vi "Write Selection.vi"(8 "error in (no error)":errorcluster, 10 "Select Tags[]":string[](array[string]), 11 "TreeSelectionHierarchal in":refnum<class "TreeSelectionHierarchal.lvclass">) -> (0 "error out":errorcluster, 3 "TreeSelectionHierarchal out":refnum<class "TreeSelectionHierarchal.lvclass">)   [LabVIEW 2015, in "TreeSelectionHierarchal.lvclass"]
doc: "This property gets or sets the items which are selected (have the TRUE checkbox).\n<b> </b> <b> </b>\n©2016 Q Software Innovations, LLC (QSI)\nwritten by Quentin Alldredge\nproduced in LabVIEW 2015\n\nsupport@qsoftwareinnovations.com\nwww.qsoftwareinnovations.com\n\nAll rights reserved.\n\nRedistribution and use in source and binary forms, with or without modification, are permitted provided that the following conditions are met:\n\n * Redistributions of source code must retain the above copyright notice, this list of conditions and the following disclaimer.\n * Redistributions in binary form must reproduce the above copyright notice, this list of conditions and the following disclaimer in the documentation and/or other materials provided with the distribution.\n * Neither the name of Q Software Innovations, LLC. nor the names of its contributors may be used to endorse or promote products derived from this software without specific prior written permission.\n\nTHIS SOFTWARE IS PROVIDED BY THE COPYRIGHT HOLDERS AND CONTRIBUTORS \"AS IS\" AND ANY EXPRESS OR IMPLIED WARRANTIES, INCLUDING, BUT NOT LIMITED TO, THE IMPLIED WARRANTIES OF MERCHANTABILITY AND FITNESS FOR A PARTICULAR PURPOSE ARE DISCLAIMED. IN NO EVENT SHALL THE COPYRIGHT OWNER OR CONTRIBUTORS BE LIABLE FOR ANY DIRECT, INDIRECT, INCIDENTAL, SPECIAL, EXEMPLARY, OR CONSEQUENTIAL DAMAGES (INCLUDING, BUT NOT LIMITED TO, PROCUREMENT OF SUBSTITUTE GOODS OR SERVICES; LOSS OF USE, DATA, OR PROFITS; OR BUSINESS INTERRUPTION) HOWEVER CAUSED AND ON ANY THEORY OF LIABILITY, WHETHER IN CONTRACT, STRICT LIABILITY, OR TORT (INCLUDING NEGLIGENCE OR OTHERWISE) ARISING IN ANY WAY OUT OF THE USE OF THIS SOFTWARE, EVEN IF ADVISED OF THE POSSIBILITY OF SUCH DAMAGE."
uses:
  TreeSelectionHierarchal.lvclass
  TreeSelection/TreeSelection.lvclass
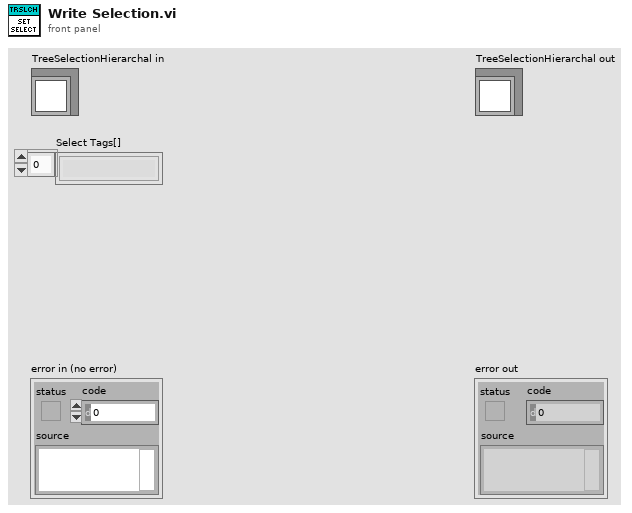
[diagram p1: front panel]
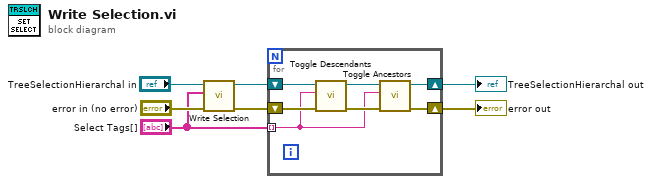
[diagram p0: block diagram]
diagram:
  n1 = call-parent "Write Selection.vi"("error in (no error)"="error in (no error)", "Selection[]"="Select Tags[]", "TreeSelection in"="TreeSelectionHierarchal in") -> ("error out"=w3:errorcluster, "TreeSelection out"=w5:refnum<class "TreeSelectionHierarchal.lvclass">)  [unwired: 7 in]
  n2 = for {
    shift-right: [w9] -> w4
    shift-left: w5 -> [w14]
    shift-right: [w11] -> w2
    shift-left: w3 -> [w13]
    tunnel: "Select Tags[]" -> [w8] mode=indexing
    n3 = call "Toggle Descendants.vi"("error in (no error)"=w13, "Tag"=w8, "TreeHier in"=w14) -> ("error out"=w12:errorcluster, "TreeHier out"=w10:refnum<class "TreeSelectionHierarchal.lvclass">)  [unwired: 7 in]
    n4 = call "Toggle Ancestors.vi"("error in (no error)"=w12, "Tag"=w8, "TreeHier in"=w10) -> ("error out"=w11:errorcluster, "TreeHier out"=w9:refnum<class "TreeSelectionHierarchal.lvclass">)  [unwired: 7 in]
  }
  "error out" <- w2
  "TreeSelectionHierarchal out" <- w4
